vi "Data From RT.vi"(0 "Queue Ref":T1, 1 "Data in":string, 3 "error in":errorcluster) -> (10 "error out":errorcluster)   [LabVIEW 2022 SP3]
uses:
  Controls/All Queue.ctl
  Controls/All Loop Status.ctl
  Global 1.vi
panel:
  out "overflow?":bool
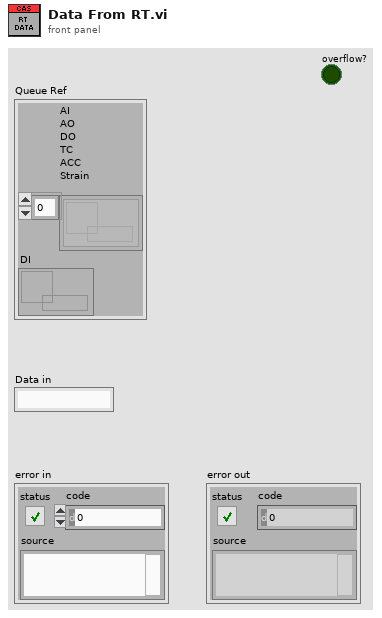
[diagram p1: front panel]
types:
  T1 = typedef "All Queue.ctl" = cluster{"AI\nAO\nDO\nTC\nACC\nStrain":refnum<queue>[], "DI":refnum<queue>}
  T2 = cluster{"AI Data":waveform(dbl)[], "AO Data":waveform(dbl)[], "DO Data":waveform(dbl)[], "TC Data":waveform(dbl)[], "ACC Data":waveform(dbl)[], "Strain Data":waveform(dbl)[], "DI Data":digitalwaveform[], "All Status":bool[], "Channel List":cluster{"AI Channel list":tag[], "AO Channel list":tag[], "DO Channel list ":tag[], "DI Channel list":tag[]}, "ALS DO":bool[], "ALS AO":dbl[], "Seq State":string}
  T3 = enum16{"Init", "Read 'All'", "Read 'n'", "Read '1'", "Write '1'", "Write 'n'", "Write 'All'"}
  T4 = typedef "All Loop Status.ctl" = enum16{"AI", "AO", "DI", "DO", "TC", "Strain", "ACC", "RT", "Log", "Seq", "Sync"}
  T5 = cluster{"AI Channel list":tag[], "AO Channel list":tag[], "DO Channel list ":tag[], "DI Channel list":tag[]}
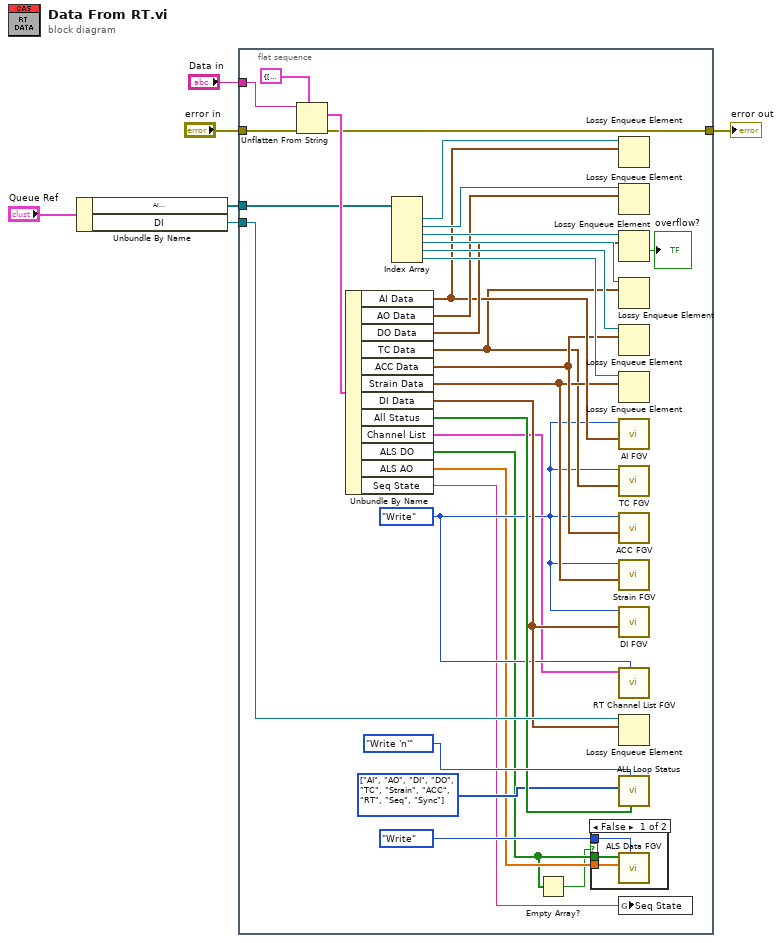
[diagram p0: block diagram]
diagram:
  n1 = Unbundle By Name("Queue Ref") -> ("AI\nAO\nDO\nTC\nACC\nStrain"=w4:refnum<queue>[], "DI"=w3:refnum<queue>)
  n2 = flat-sequence {
    tunnel: "Data in" -> [w37]
    tunnel: w4 -> [w29]
    tunnel: w3 -> [w28]
    tunnel: "error in" -> [w15]
    tunnel: [w14] -> w1
    frame #0 {
      w23 = T4[] [enum."AI", enum."AO", enum."DI", enum."DO", enum."TC", enum."Strain", enum."ACC", enum."RT", enum."Seq", enum."Sync"] items=["AI", "AO", "DI", "DO", "TC", "Strain", "ACC", "RT", "Log", "Seq", "Sync"] ("Loops")
      w17 = enum16{"Read", "Write"}."Write" ("Enum")
      n3 = Unflatten From String(type=T2 {"AI Data"=[], "AO Data"=[], "DO Data"=[], "TC Data"=[], "ACC Data"=[], "Strain Data"=[], "DI Data"=[], "All Status"=[], "Channel List"={"AI Channel list"=[], "AO Channel list"=[], "DO Channel list "=[], "DI Channel list"=[]}, "ALS DO"=[], "ALS AO"=[], "Seq State"=""}, binary string=w37, error in (no error)=w15) -> (value=w30:T2, error out=w14:errorcluster)  [unwired: 2 in, 1 out]
      n4 = Unbundle By Name(w30) -> ("AI Data"=w22:waveform(dbl)[], "AO Data"=w27:waveform(dbl)[], "DO Data"=w26:waveform(dbl)[], "TC Data"=w18:waveform(dbl)[], "ACC Data"=w21:waveform(dbl)[], "Strain Data"=w20:waveform(dbl)[], "DI Data"=w19:digitalwaveform[], "All Status"=w24:bool[], "Channel List"=w16:T5, "ALS DO"=w9:bool[], "ALS AO"=w11:dbl[], "Seq State"=w10:string)
      n5 = Index Array(array=w29) -> (element #1=w36:refnum<queue>, element #2=w35:refnum<queue>, element #3=w34:refnum<queue>, element #4=w33:refnum<queue>, element #5=w32:refnum<queue>, element #6=w31:refnum<queue>)  [unwired: 6 in]
      n6 = Empty Array?(array=w9) -> (empty?=w8:bool)
      n7 = case shown="False" w8 {
        tunnel: enum16{"Read", "Write"}."Write" ("Enum") -> [w40 _]
        tunnel: w9 -> [w39 _]
        tunnel: w11 -> [w38 _]
        frame False {
          n8 = call "ALS Data FGV.vi"("Enum"=w40, "ALS AO in"=w38, "ALS DO in"=w39) -> ()  [unwired: 6 in, 3 out]
        }
        frame True {
        }
      }
      n9 = Lossy Enqueue Element(queue=w36, element=w22) -> ()  [unwired: 1 in, 4 out]
      n10 = Lossy Enqueue Element(queue=w35, element=w27) -> ()  [unwired: 1 in, 4 out]
      n11 = Lossy Enqueue Element(queue=w34, element=w26) -> (overflow?=→"overflow?":bool)  [unwired: 1 in, 3 out]
      n12 = Lossy Enqueue Element(queue=w33, element=w18) -> ()  [unwired: 1 in, 4 out]
      n13 = Lossy Enqueue Element(queue=w32, element=w21) -> ()  [unwired: 1 in, 4 out]
      n14 = Lossy Enqueue Element(queue=w31, element=w20) -> ()  [unwired: 1 in, 4 out]
      n15 = call "AI FGV.vi"("AI data"=w22, "Enum"=w17) -> ()  [unwired: 9 in, 1 out]
      n16 = call "TC FGV.vi"("AI data"=w18, "Enum"=w17) -> ()  [unwired: 9 in, 1 out]
      n17 = call "ACC FGV.vi"("AI data"=w21, "Enum"=w17) -> ()  [unwired: 9 in, 1 out]
      n18 = call "Strain FGV.vi"("AI data"=w20, "Enum"=w17) -> ()  [unwired: 9 in, 1 out]
      n19 = call "DI FGV.vi"("DI Data"=w19, "Enum"=w17) -> ()  [unwired: 9 in, 1 out]
      n20 = call "RT Channel List FGV.vi"("Enum"=w17, "Channel List in"=w16) -> ()  [unwired: 8 in, 2 out]
      n21 = Lossy Enqueue Element(queue=w28, element=w19) -> ()  [unwired: 1 in, 4 out]
      n22 = call "ALL Loop Status.vi"("Status List"=w24, "Option"=T3."Write 'n'", "Loops"=w23) -> ()  [unwired: 6 in, 3 out]
      n23 = global write "Global 1.vi" "Seq State"(w10) -> ()
    }
  }
  "error out" <- w1
